vi "Handle Error.vi"(8 "error in (no error)":errorcluster, 11 "Async Methods Actor Example in":refnum<class "Async Methods Actor Example.lvclass">) -> (0 "error out":errorcluster, 2 "stop actor?":bool=TRUE, 3 "Async Methods Actor Example out":refnum<class "Async Methods Actor Example.lvclass">)   [LabVIEW 2023, in "Async Methods Actor Example.lvlib" / "Async Methods Actor Example.lvclass"]
doc: "(<B>Filename</B>: Actor Framework.lvlib:Actor.lvclass:Handle Error.vi)\n\nDefines how the actor handles an error that occurred while processing a message. By default, this method does nothing except stop the actor."
uses:
  Async Methods Actor Example.lvclass
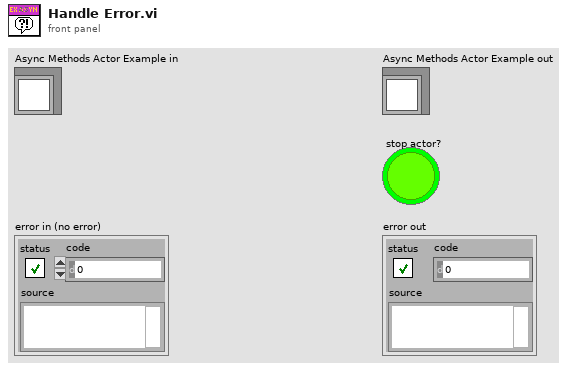
[diagram p1: front panel]
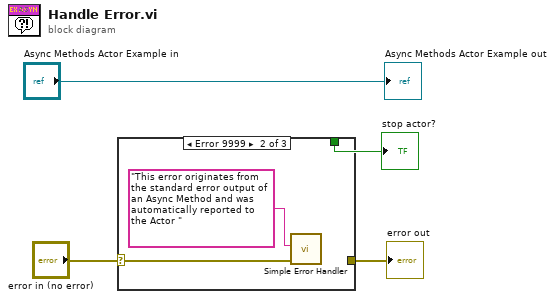
[diagram p0: block diagram]
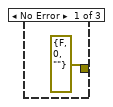
[diagram p2: hidden frame]
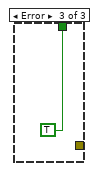
[diagram p3: hidden frame]
diagram:
  n1 = case shown="Error 9999" "error in (no error)" {
    selector: "error in (no error)" -> [_ w7 _]
    tunnel: [errorcluster {"status"=FALSE, "code"=0, "source"=""} ("error out") _ _] -> w2
    tunnel: [_ _ TRUE ("stop actor?")] -> w1
    frame No Error {
    }
    frame Error {
      n2 = call <vilib>:"Simple Error Handler.vi"("error source (\" \")"="This error originates from the standard error output of an Async Method and was automatically reported to the Actor " ("error source (\" \")"), "error in (no error)"=w7) -> ()  [unwired: 3 in, 5 out]
    }
    frame Error {
    }
  }
  "error out" <- w2
  "stop actor?" <- w1
  "Async Methods Actor Example out" <- "Async Methods Actor Example in"
